vi "test_write_key_integer.vi"(8 "error in (no error)":errorcluster) -> (0 "error out":errorcluster)   [LabVIEW 2020]
uses:
  toml/toml.lvclass
  <vilib>/addons/_JKI Toolkits/Caraya/classes/Assert/Assert.lvclass
  <vilib>/addons/_JKI Toolkits/Caraya/classes/Test/Test.lvclass
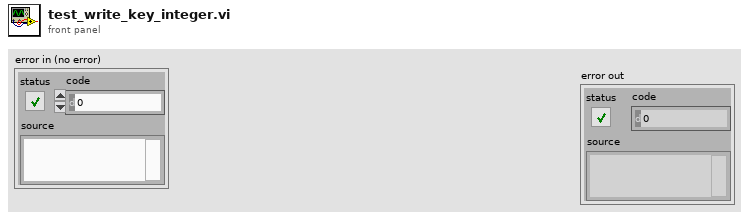
[diagram p1: front panel]
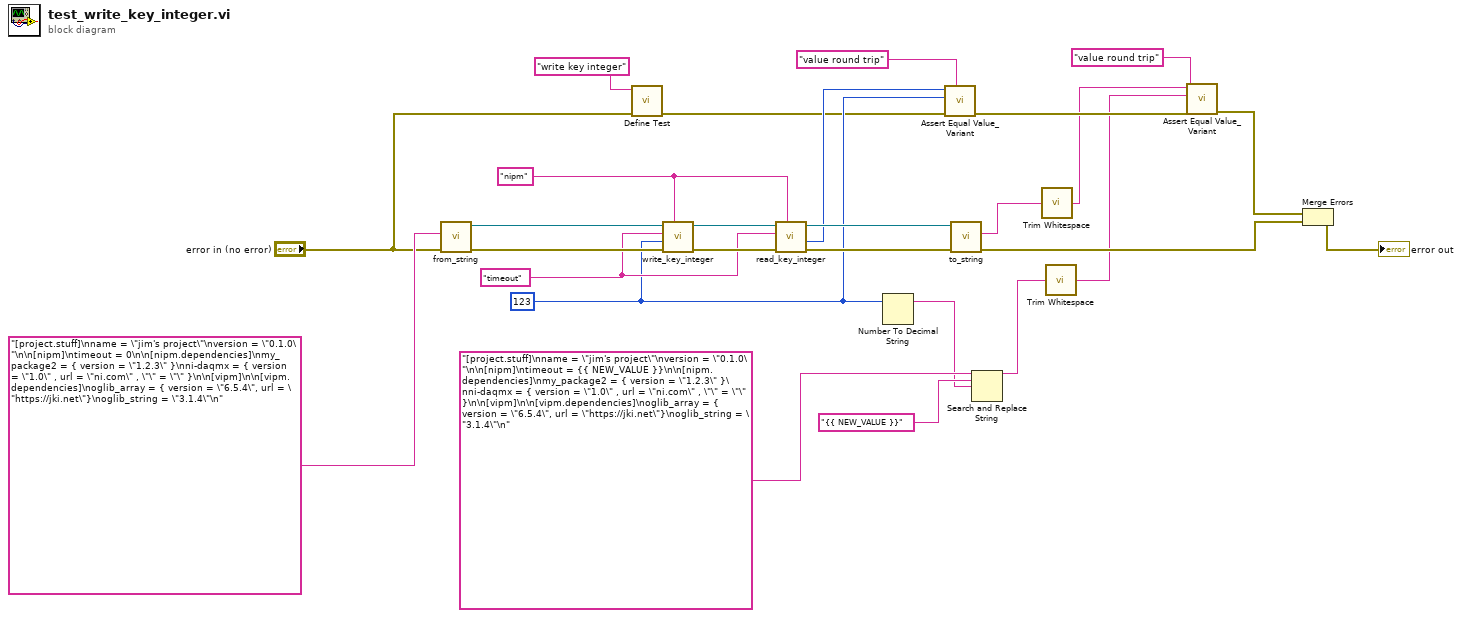
[diagram p0: block diagram]
diagram:
  w19 = "timeout" ("table_name")
  w20 = "nipm" ("table_name")
  w9 = 123 ("string")
  n1 = call "from_string.vi"("error in (no error)"="error in (no error)", "toml"="[project.stuff]\nname = \"jim's project\"\nversion = \"0.1.0\"\n\n[nipm]\ntimeout = 0\n\n[nipm.dependencies]\nmy_package2 = { version = \"1.2.3\" }\nni-daqmx = { version = \"1.0\" , url = \"ni.com\" , \"\" = \"\" }\n\n[vipm]\n\n[vipm.dependencies]\noglib_array = { version = \"6.5.4\", url = \"https://jki.net\"}\noglib_string = \"3.1.4\"\n" ("toml_string in")) -> ("error out"=w22:errorcluster, "toml out"=w21:refnum<class "toml.lvclass">)  [unwired: 8 in]
  n2 = call <vilib>:"Define Test.vi"("error in (no error)"="error in (no error)", "Label (VI Title)"="write key integer") -> ("error out"=w7:errorcluster)  [unwired: 9 in]
  n3 = call "write_key_integer.vi"("table"=w20, "error in (no error)"=w22, "value"=w9, "key"=w19, "toml in"=w21) -> ("error out"=w26:errorcluster, "toml out"=w24:refnum<class "toml.lvclass">)  [unwired: 5 in]
  n4 = call "read_key_integer.vi"("table"=w20, "error in (no error)"=w26, "key"=w19, "toml in"=w24) -> ("error out"=w25:errorcluster, "value"=w18:i64, "toml out"=w23:refnum<class "toml.lvclass">)  [unwired: 5 in]
  n5 = Number To Decimal String(number=w9) -> (decimal integer string=w1:string)  [unwired: 1 in]
  n6 = call <vilib>:"Assert Equal Value_Variant.vi"("Label"="value round trip", "error in (no error)"=w7, "Y"=w9, "X"=w18) -> ("error out"=w17:errorcluster)  [unwired: 7 in]
  n7 = call "to_string.vi"("error in (no error)"=w25, "toml in"=w23) -> ("error out"=w14:errorcluster, "toml_string"=w5:string)  [unwired: 8 in]
  n8 = Search and Replace String(input string="[project.stuff]\nname = \"jim's project\"\nversion = \"0.1.0\"\n\n[nipm]\ntimeout = {{ NEW_VALUE }}\n\n[nipm.dependencies]\nmy_package2 = { version = \"1.2.3\" }\nni-daqmx = { version = \"1.0\" , url = \"ni.com\" , \"\" = \"\" }\n\n[vipm]\n\n[vipm.dependencies]\noglib_array = { version = \"6.5.4\", url = \"https://jki.net\"}\noglib_string = \"3.1.4\"\n" ("toml_string in"), search string="{{ NEW_VALUE }}", replace string=w1) -> (result string=w3:string)  [unwired: 5 in, 3 out]
  n9 = call <vilib>:"Trim Whitespace.vi"("string"=w5) -> ("trimmed string"=w4:string)  [unwired: 1 in]
  n10 = call <vilib>:"Trim Whitespace.vi"("string"=w3) -> ("trimmed string"=w2:string)  [unwired: 1 in]
  n11 = call <vilib>:"Assert Equal Value_Variant.vi"("Label"="value round trip", "error in (no error)"=w17, "Y"=w2, "X"=w4) -> ("error out"=w15:errorcluster)  [unwired: 7 in]
  n12 = Merge Errors(w15, w14) -> (→"error out":errorcluster)
